vi "stringToBase64.vi"(1 "Original":string) -> (0 "Base 64":string)   [LabVIEW 2012]
uses:
  C:/Documents and Settings/Administrator/Desktop/alpha-push-dll-0.1.1-SNAPSHOT/lib/IKVM.OpenJDK.Core.dll
  \\VBOXSVR\labview-java-example/commons-codec-dll/target/Apache.Commons.Codec.dll
  commons-codec-dll/target/Apache.Commons.Codec.dll
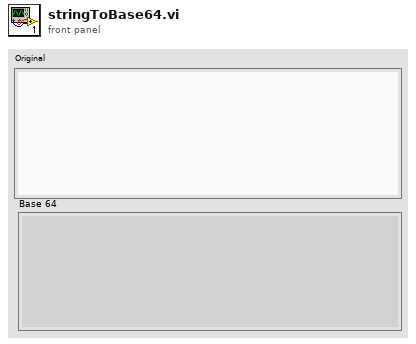
[diagram p1: front panel]
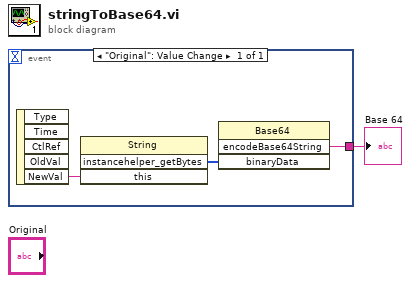
[diagram p0: block diagram]
diagram:
  n1 = event shown="[0] \"Original\": Value Change" {
    selector: _ -> [_]
    dyn-events: _ -> [_]
    timeout: _ -> [_]
    tunnel: [w2] -> w1
    event "Original": Value Change {
      n2 = event-data() -> ("NewVal"=w3:string)  [unwired: 1 in, 4 out]
      n3 = invoke class="String" method="instancehelper_getBytes"("this"=w3) -> ("instancehelper_getBytes"=w4:u8[])  [unwired: 3 in, 3 out]
      n4 = invoke class="Base64" method="encodeBase64String"("binaryData"=w4) -> ("encodeBase64String"=w2:string)  [unwired: 3 in, 3 out]
    }
  }
  "Base 64" <- w1
